vi "EnableVelocityWindow.vi"(4 "error in (no error)":errorcluster, 6 "velocity window":T1, 7 "axis in":cluster{"keyHandle":u32, "nodeId":u16}={"keyHandle"=0, "nodeId"=1}) -> (0 "error out":errorcluster, 3 "axis out":cluster{"keyHandle":u32, "nodeId":u16}={"keyHandle"=0, "nodeId"=1})   [LabVIEW 2017, in "maxonEPOS.lvlib"]
doc: "<B>EnableVelocityWindow</B> activates the velocity window."
uses:
  Examples/maxonEPOS.lvlib
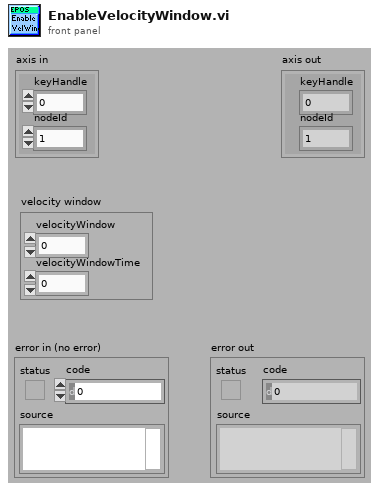
[diagram p1: front panel]
types:
  T1 = cluster{"velocityWindow":u32, "velocityWindowTime":u16}
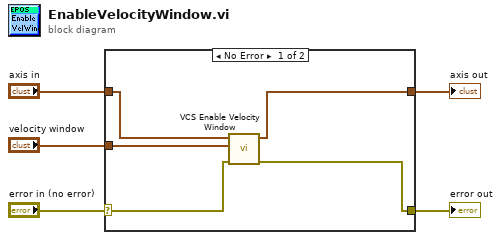
[diagram p0: block diagram]
diagram:
  n1 = case shown="No Error" "error in (no error)" {
    selector: "error in (no error)" -> [w6 w12]
    tunnel: [w7 w12] -> w4
    tunnel: [w8 w11] -> w3
    tunnel: "axis in" -> [w9 w11]
    tunnel: "velocity window" -> [w10 _]
    frame No Error {
      n2 = call "VCS Enable Velocity Window.vi"("error in (no error)"=w6, "velocity window"=w10, "axis in"=w9) -> ("error out"=w7:errorcluster, "axis out"=w8:cluster{"keyHandle":u32, "nodeId":u16})  [unwired: 7 in]
    }
    frame Error {
    }
  }
  "error out" <- w4
  "axis out" <- w3
